vi "main_NoMotion.vi"() -> ()   [LabVIEW 2023]
panel:
  out "Tx Sampling Rate":dbl
  out "End Frequency":dbl
  out "Start Frequency":dbl
  out "Tx Duration":dbl
  in  "Group Delay":dbl
  out "Tx Waveform":waveform(dbl)(graph)
  out "Rx Data":waveform(dbl)[](graph)
  in  "Tx Amplitude":dbl=1.0 format="%0.2p"
  in  "AO Trigger Source":tag
  in  "DAQmx Device Name":tag
  in  "Rx Sampling Rate":dbl
  in  "Rx Duration":dbl
  in  "Voltage Rails":dbl
  in  "Data Export Path":path
  in  "Waveform Input Path":path
  out "error out":errorcluster
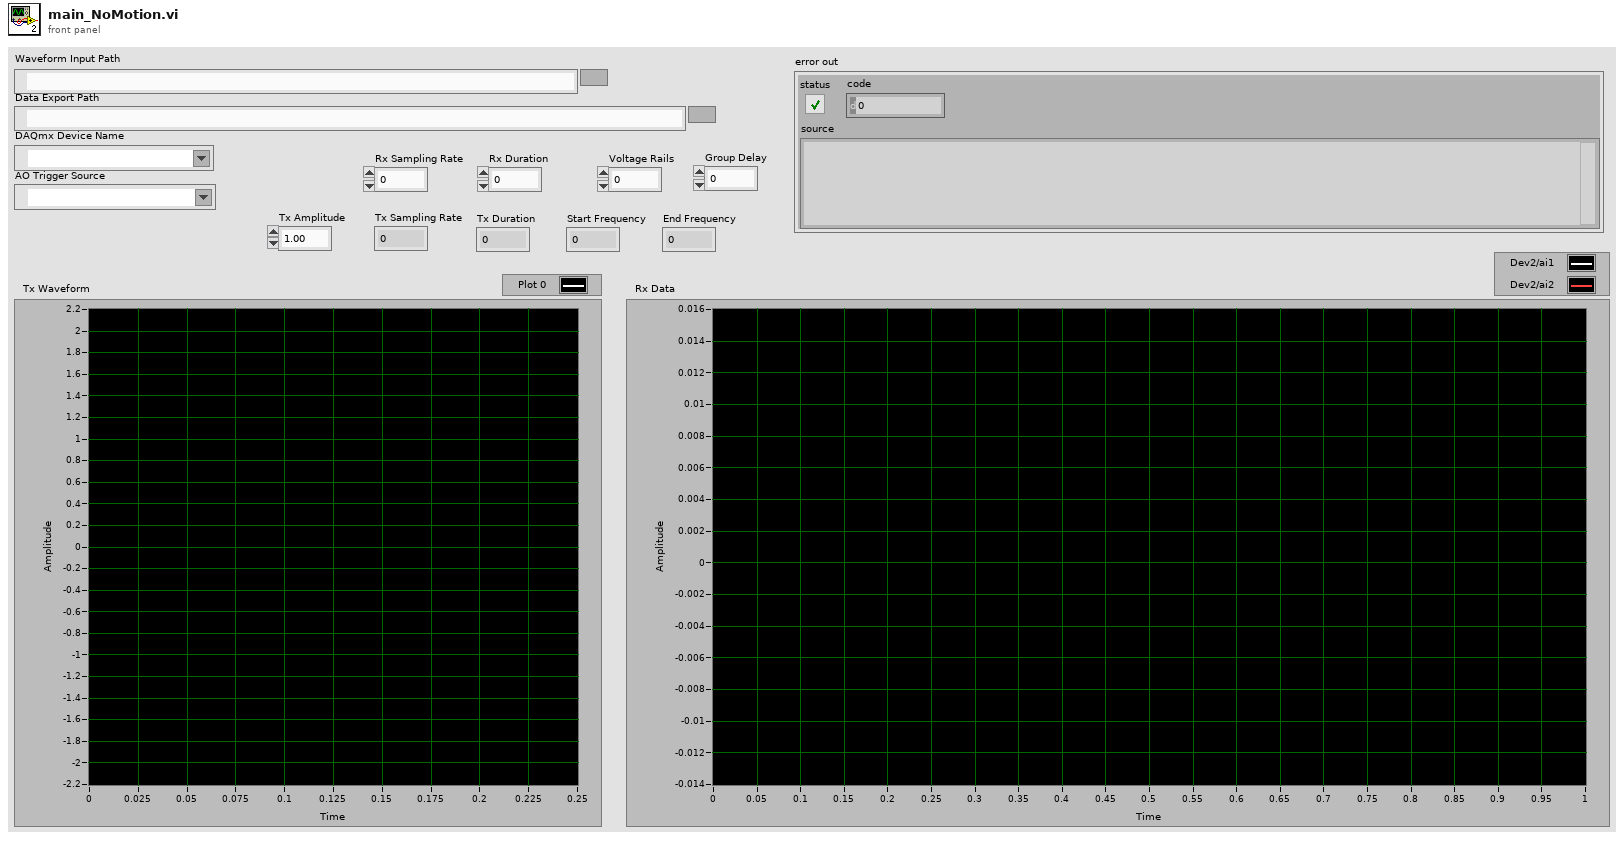
[diagram p1: front panel]
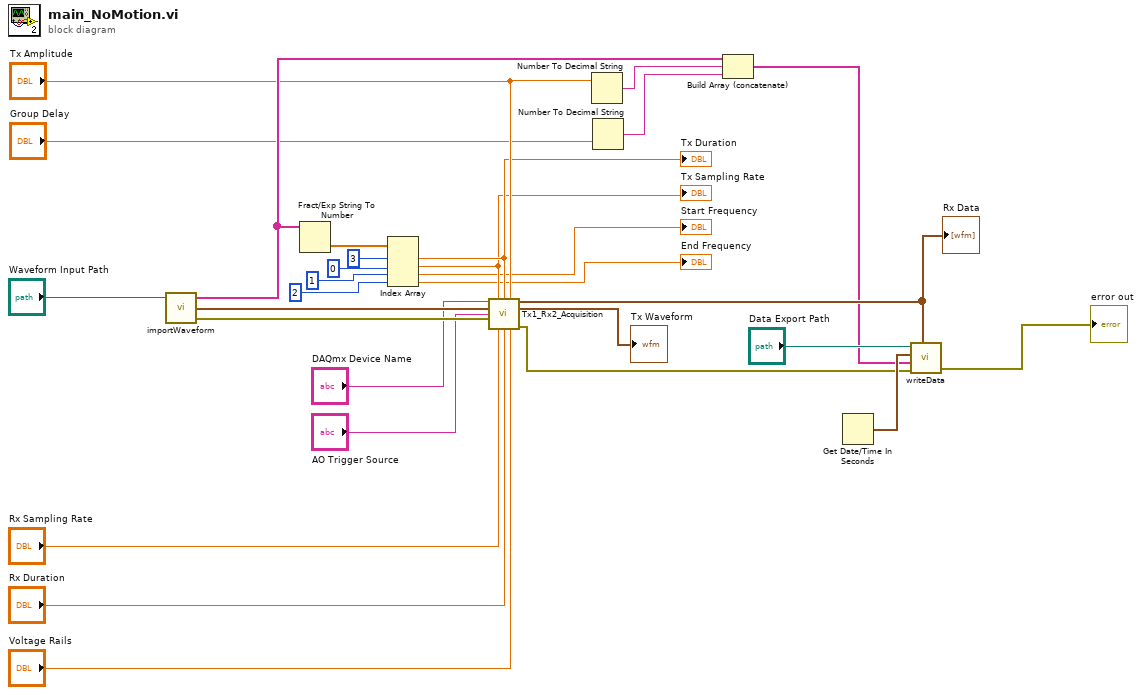
[diagram p0: block diagram]
diagram:
  n1 = call "importWaveform.vi"("Path to Waveform"="Waveform Input Path") -> ("error out"=w22:errorcluster, "output waveform"=w21:waveform(dbl), "Params"=w12:string[])  [unwired: 2 in]
  n2 = Fract/Exp String To Number(string=w12) -> (number=w18:dbl[])  [unwired: 3 in, 1 out]
  n3 = Index Array(array=w18, index #1=3 ("index"), index #2=0 ("index"), index #3=1 ("index"), index #4=2 ("index")) -> (element #1=w4:dbl, element #2=w3:dbl, element #3=→"Start Frequency":dbl, element #4=→"End Frequency":dbl)
  "Tx Duration" <- w4
  "Tx Sampling Rate" <- w3
  n4 = call "Tx1_Rx2_Acquisition.vi"("DAQmx Device Name"="DAQmx Device Name", "Tx Sampling Rate"=w3, "Transmit Duration"=w4, "Tx Amplitude"="Tx Amplitude", "Tx Waveform"=w21, "AO Trigger Source"="AO Trigger Source", "error in"=w22, "Rx Sampling Rate"="Rx Sampling Rate", "Receive Duration"="Rx Duration", "Voltage Rails"="Voltage Rails") -> ("Rx Data"=w15:waveform(dbl)[], "Tx Waveform"=→"Tx Waveform":waveform(dbl), "error out"=w13:errorcluster)  [unwired: 3 in]
  "Rx Data" <- w15
  n5 = Number To Decimal String(number="Tx Amplitude") -> (decimal integer string=w11:string)  [unwired: 1 in]
  n6 = Number To Decimal String(number="Group Delay") -> (decimal integer string=w9:string)  [unwired: 1 in]
  n7 = Build Array (concatenate)(w12, w11, w9) -> (w7:string[])
  n8 = Get Date/Time In Seconds() -> (seconds since 1Jan1904=w27:timestamp)
  n9 = call "writeData.vi"("base path"="Data Export Path", "time stamp"=w27, "Parameters"=w7, "error in"=w13, "Input data"=w15) -> ("error out"=→"error out":errorcluster)  [unwired: 2 in]
